vi "Write move waveplate.vi"(8 "error in (no error)":errorcluster, 10 "move waveplate":bool, 11 "Sim_Ixon_Ultra in":refnum<class "Sim_Ixon_Ultra.lvclass">) -> (0 "error out":errorcluster, 3 "Sim_Ixon_Ultra out":refnum<class "Sim_Ixon_Ultra.lvclass">)   [LabVIEW 2018, in "Sim_Ixon_Ultra.lvclass"]
uses:
  Sim_Ixon_Ultra.lvclass
  Sim_Ixon_Ultra.lvclass/Sim_Ixon_Ultra.ctl
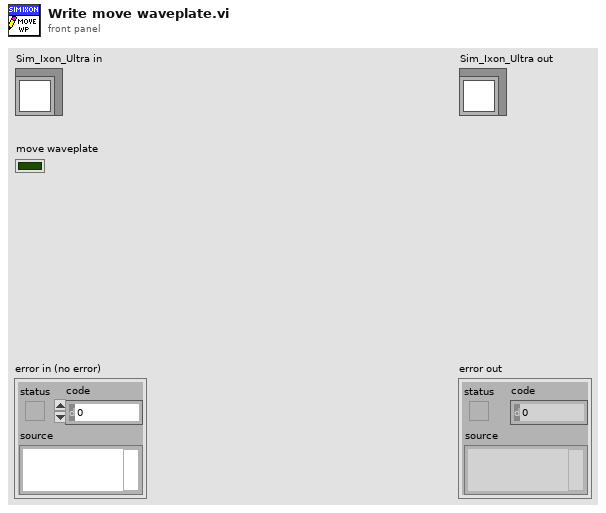
[diagram p1: front panel]
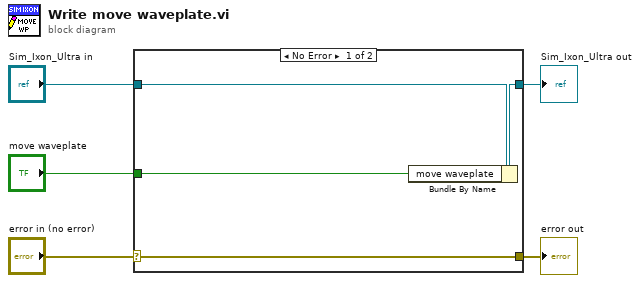
[diagram p0: block diagram]
diagram:
  n1 = case shown="No Error" "error in (no error)" {
    selector: "error in (no error)" -> [w9 w10]
    tunnel: [w9 w10] -> w4
    tunnel: [w7 w11] -> w2
    tunnel: "Sim_Ixon_Ultra in" -> [w8 w11]
    tunnel: "move waveplate" -> [w6 _]
    frame No Error {
      n2 = Bundle By Name(cluster=w8, "move waveplate"=w6) -> (w7:refnum<class "Sim_Ixon_Ultra.lvclass">)
    }
    frame Error {
    }
  }
  "error out" <- w4
  "Sim_Ixon_Ultra out" <- w2
